vi "calcForceCoefficient.vi"(8 "error in (no error)":errorcluster, 11 "ForceSensor in":refnum<class "ForceSensorCalculator.lvclass">) -> (0 "error out":errorcluster, 3 "ForceSensor out":refnum<class "ForceSensorCalculator.lvclass">)   [LabVIEW 2013, in "ForceSensorCalculator.lvlib" / "ForceSensorCalculator.lvclass"]
uses:
  <userlib>/Common/Devices/ForceSensorCalculator/ForceSensorCalculator/ForceSensorCalculator.lvclass
  <userlib>/Common/Devices/ForceSensorCalculator/ForceSensorCalculator/ForceSensorCalculator.lvclass/ForceSensorCalculator.ctl
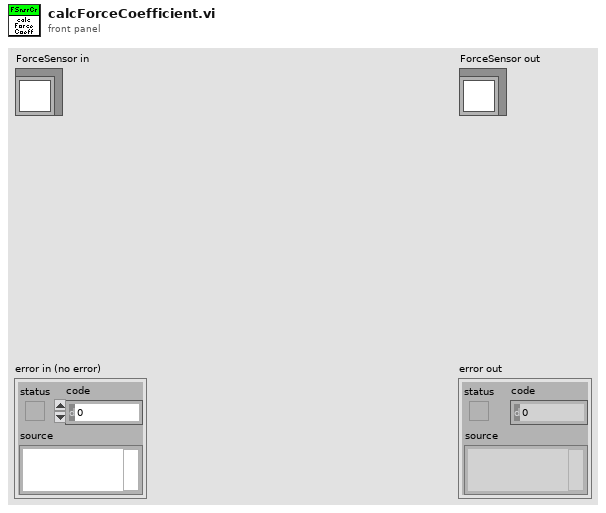
[diagram p1: front panel]
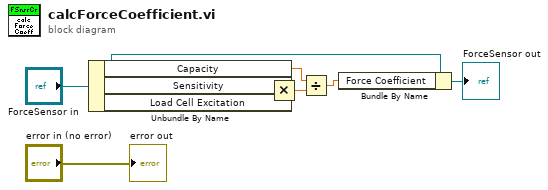
[diagram p0: block diagram]
diagram:
  n1 = Unbundle By Name("ForceSensor in") -> ("Capacity"=w6:dbl[unit], "Sensitivity"=w8:dbl[unit], "Load Cell Excitation"=w7:dbl[unit])
  n2 = Multiply(x=w8, y=w7) -> (x*y=w5:dbl[unit])
  n3 = Divide(x=w6, y=w5) -> (x/y=w4:dbl[unit])
  n4 = Bundle By Name(cluster="ForceSensor in", "Force Coefficient"=w4) -> (→"ForceSensor out":refnum<class "ForceSensorCalculator.lvclass">)
  "error out" <- "error in (no error)"
